vi "SaveWWWChartImages.vi"(9 "Chart Refs":refnum<vi>[](array[refnum]), 10 "Destination":path, 11 "VI in":refnum<vi>) -> ()   [LabVIEW 2017]
panel:
  out "Write Imegtime":u32
  out "get Imegtime":u32
  out "Time":u32
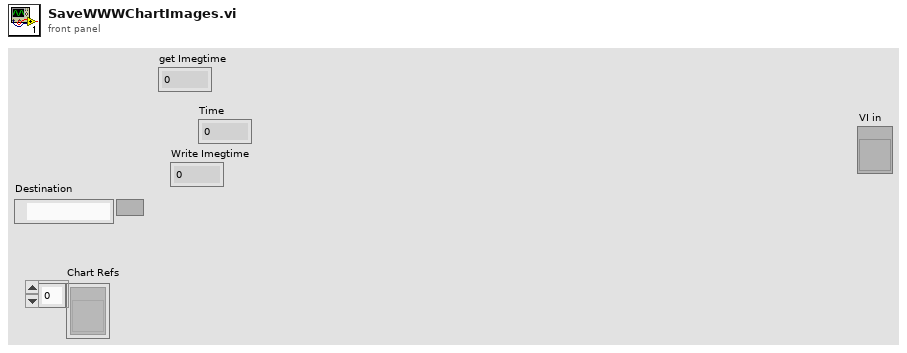
[diagram p1: front panel]
types:
  T1 = typedef "imagedata.ctl" = cluster{"image type":i32, "image depth":i32, "image":u8[], "mask":u8[], "colors":u32[], "Rectangle":cluster{"left":i16, "top":i16, "right":i16, "bottom":i16}}
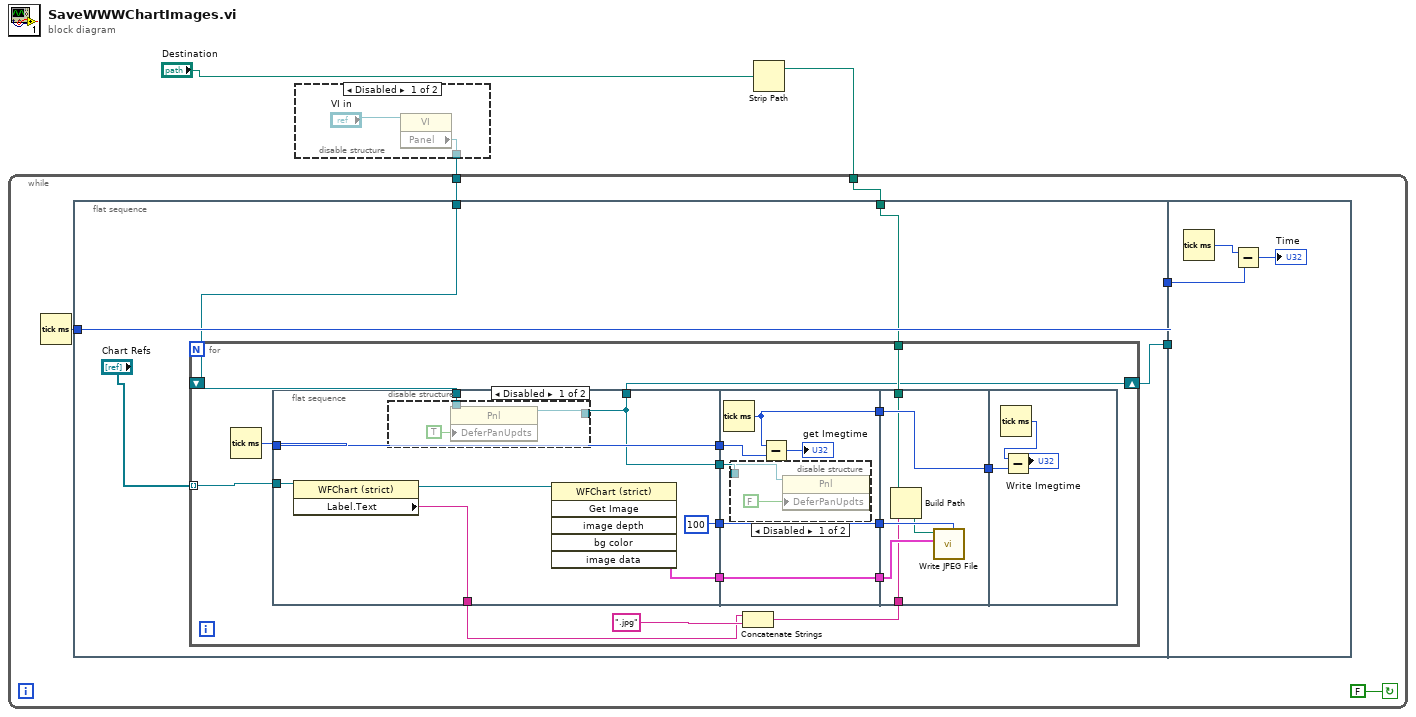
[diagram p0: block diagram]
diagram:
  n1 = disable-structure shown="Disabled" {
    disable-tunnel: [w4 _] -> w1
    frame Disabled {
      n2 = property class="VI"(reference="VI in") -> ("Panel"=w4:refnum<vi>)  [unwired: 1 in, 2 out]
    }
    frame Enabled {
    }
  }
  n3 = Strip Path(path="Destination") -> (stripped path=w2:path)  [unwired: 1 out]
  n4 = while {
    tunnel: w2 -> [w7]
    tunnel: w1 -> [w6]
    stop <- FALSE continue-if-true
    n5 = Tick Count (ms)() -> (millisecond timer value=w9:u32)
    n6 = flat-sequence {
      tunnel: [w13] -> w11
      tunnel: [w16] -> w10
      tunnel: w9 -> [w16]
      tunnel: w7 -> [w15]
      tunnel: w6 -> [w14]
      tunnel: w11 -> [_]
      tunnel: w10 -> [w62]
      frame #0 {
        n7 = for {
          tunnel: w15 -> [w24]
          shift-right: [w22] -> w13
          shift-left: w14 -> [w23]
          tunnel: "Chart Refs" -> [w17] mode=indexing
          n8 = Tick Count (ms)() -> (millisecond timer value=w20:u32)
          n9 = flat-sequence {
            tunnel: w17 -> [w40]
            tunnel: [w38] -> w32
            tunnel: [100 ("quality (80)")] -> w31
            tunnel: [w36] -> w30
            tunnel: w20 -> [w36]
            tunnel: [w33] -> w19
            tunnel: w23 -> [w35]
            tunnel: [w34] -> w22
            tunnel: [w34] -> w29
            tunnel: w32 -> [w49]
            tunnel: [w49] -> w28
            tunnel: w31 -> [w48]
            tunnel: [w48] -> w27
            tunnel: w30 -> [w47]
            tunnel: [w45] -> w26
            tunnel: w29 -> [w44]
            tunnel: w28 -> [w56]
            tunnel: w27 -> [w57]
            tunnel: w26 -> [w55]
            tunnel: [w55] -> w25
            tunnel: w24 -> [w54]
            tunnel: w18 -> [w52]
            tunnel: w25 -> [w58]
            frame #0 {
              n10 = property class="WFChart (strict)"(reference=w40) -> (reference out=w39:refnum<vi>, "Label.Text"=w33:string)  [unwired: 1 in, 1 out]
              n11 = disable-structure shown="Disabled" {
                disable-tunnel: w35 -> [w43 _]
                disable-tunnel: [w41 _] -> w34
                frame Disabled {
                  n12 = property class="Pnl"(reference=w43, "DeferPanUpdts"=TRUE ("Defer Panel Updates")) -> (reference out=w41:refnum<vi>)  [unwired: 1 in, 1 out]
                }
                frame Enabled {
                }
              }
              n13 = invoke class="WFChart (strict)" method="Get Image"(reference=w39) -> ("image data"=w38:T1)  [unwired: 5 in, 5 out]
            }
            frame #1 {
              n14 = Tick Count (ms)() -> (millisecond timer value=w45:u32)
              n15 = disable-structure shown="Disabled" {
                disable-tunnel: w44 -> [w50 _]
                frame Disabled {
                  n16 = property class="Pnl"(reference=w50, "DeferPanUpdts"=FALSE ("Defer Panel Updates")) -> ()  [unwired: 1 in, 2 out]
                }
                frame Enabled {
                }
              }
              n17 = Subtract(x=w45, y=w47) -> (x-y=→"get Imegtime":u32)
            }
            frame #2 {
              n18 = Build Path(base path=w54, name or relative path=w52) -> (appended path=w53:path)
              n19 = call <vilib>:"Write JPEG File.vi"("quality (80)"=w57, "image data"=w56, "path to JPEG file"=w53) -> ()  [unwired: 7 in, 2 out]
            }
            frame #3 {
              n20 = Tick Count (ms)() -> (millisecond timer value=w59:u32)
              n21 = Subtract(x=w59, y=w58) -> (x-y=→"Write Imegtime":u32)
            }
          }
          n22 = Concatenate Strings(w19, ".jpg" ("string")) -> (w18:string)
        }
      }
      frame #1 {
        n23 = Tick Count (ms)() -> (millisecond timer value=w63:u32)
        n24 = Subtract(x=w63, y=w62) -> (x-y=→"Time":u32)
      }
    }
  }
